vi "FRCts20_EspEngine_ConvertToEvent.vi"() -> ()   [LabVIEW 2013, in "FRCts20_EspEngine.lvlib"]
uses:
  FRCts20_EspEngine.lvlib
  Web Methods/source/VI Source/Web Method Public Interface/FRCts20_WebMethods_ctl_teamIdentifier.ctl
  Web Methods/source/VI Source/FRCts20_WebMethods.lvlib
  Web Methods/source/VI Source/Web Method Public Interface/FRCts20_WebMethods_ctl_events.ctl
  Web Methods/source/VI Source/Web Method Public Interface/FRCts20_WebMethods_ctl_singleEvent.ctl
panel:
  in  "Events":T1
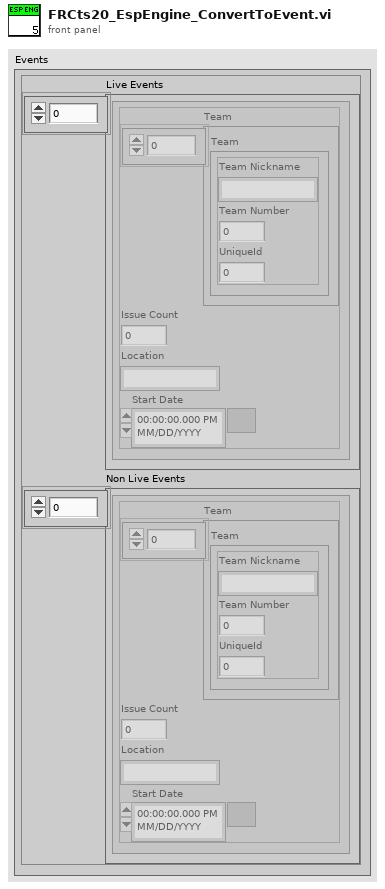
[diagram p1: front panel]
types:
  T1 = typedef "FRCts20_WebMethods.lvlib/FRCts20_WebMethods_ctl_events.ctl" = cluster{"Live Events":cluster{"Team":T2[], "Issue Count":i32, "Location":string, "Start Date ":timestamp}[], "Non Live Events":T3[]}
  T2 = typedef "FRCts20_WebMethods.lvlib/FRCts20_WebMethods_ctl_teamIdentifier.ctl" = cluster{"Team Nickname":string, "Team Number ":u32, "UniqueId":u32}
  T3 = typedef "FRCts20_WebMethods.lvlib/FRCts20_WebMethods_ctl_singleEvent.ctl" = cluster{"Team":T2[], "Issue Count":i32, "Location":string, "Start Date ":timestamp}
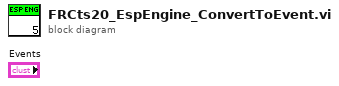
[diagram p0: block diagram]
diagram:
